vi "Target CSM.vi"(5 "Init State(\"Macro: Initialize\")":string="Macro: Initialize", 7 "Name(\"\" to use uuid)":string="CSM Tiny") -> ()   [LabVIEW 2017]
doc: "Template for building CSM Module without User Interface.\n\n<b>Inputs:</b>\n- <b>Name(\"\" to use uuid)</b>: Module Name\n - If Input is \"\", an uuid will be used for module name. The module is marked as stand-alone mode and will not be included in module list.\n - Fi Input end with '#', the module will worked in worker mode. Modules with the same name will shared the same message queue. Any external message will be processed by one of the modules, depends on who is free.\n - Otherwise, the input string will be used as module name, which should be unique in system. CSM will go to \"Critical Error\" state if duplicated module name is used in system.\n\n<b>Outputs:</b>\n - N/A"
uses:
  src/user.lib/_NEVSTOP/Communicable State Machine(CSM)/AdvanceAPI/CSM - Revert Arguments-Safe String.vi
  src/user.lib/_NEVSTOP/Communicable State Machine(CSM)/_Support/Common/Trim Single line Text.vi
  src/user.lib/_NEVSTOP/Communicable State Machine(CSM)/AdvanceAPI/CSM - Break Down Multiple States String.vi
  src/user.lib/_NEVSTOP/Communicable State Machine(CSM)/AdvanceAPI/CSM - Compact Multiple States.vi
  src/user.lib/_NEVSTOP/Communicable State Machine(CSM)/AdvanceAPI/CSM - Make String Arguments Safe.vi
  src/user.lib/_NEVSTOP/Communicable State Machine(CSM)/_Support/Common/Format Timestamp.vi
  src/user.lib/_NEVSTOP/Communicable State Machine(CSM)/AdvanceAPI/CSM - Keywords.vi
  src/user.lib/_NEVSTOP/Communicable State Machine(CSM)/Communicable State Machine.lvlib
panel:
  out "State History":string
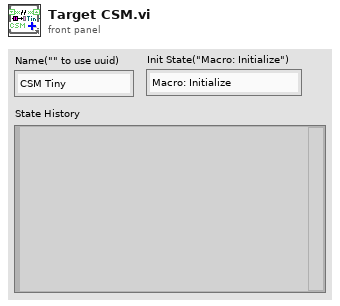
[diagram p1: front panel]
types:
  T1 = enum32{"Invalid", "Standard", "Closed", "Hidden", "Minimized", "Maximized"}
  T2 = enum32{"invalid app kind", "Development System", "Run Time System", "Student Edition", "Embedded LabVIEW", "Evaluation", "Custom"}
  T3 = typedef "Communicable State Machine.lvlib/_CSM_Response Source Message.ctl" = cluster{"‘State":string, "’Arguments":string, "’Error":errorcluster}
  T4 = cluster{"Core":cluster{"Current VI Reference":refnum<vi>, "Close Panel on Exit?":bool}, "Your Boolean data":bool, "Your string data":string}
  T5 = cluster{"Current VI Reference":refnum<vi>, "Close Panel on Exit?":bool}
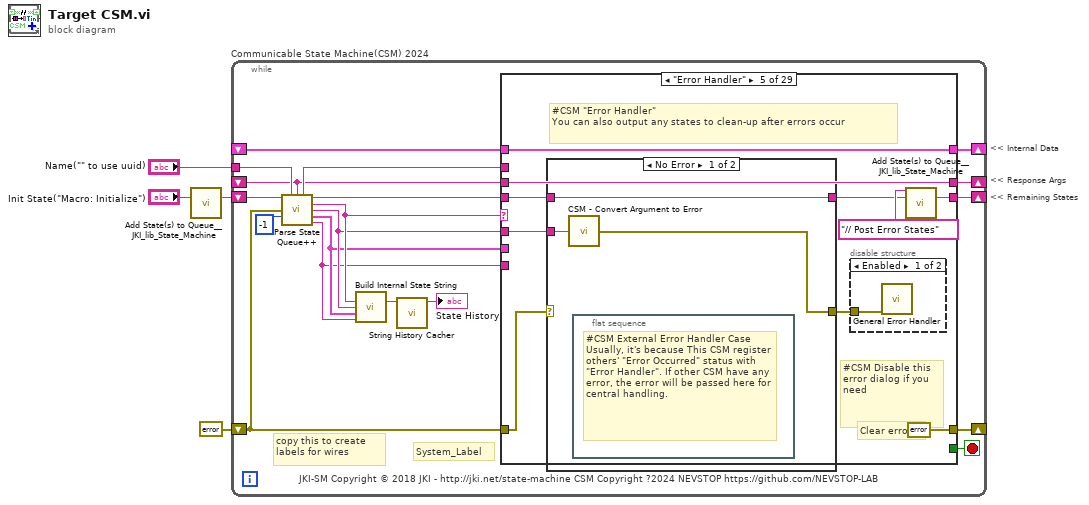
[diagram p0: block diagram]
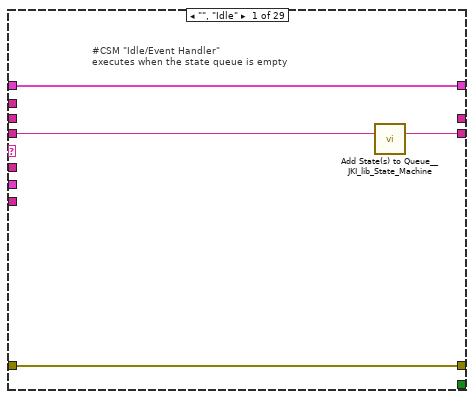
[diagram p2: hidden frame]
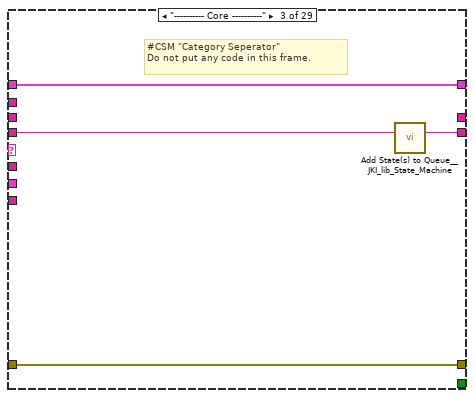
[diagram p4: hidden frame]
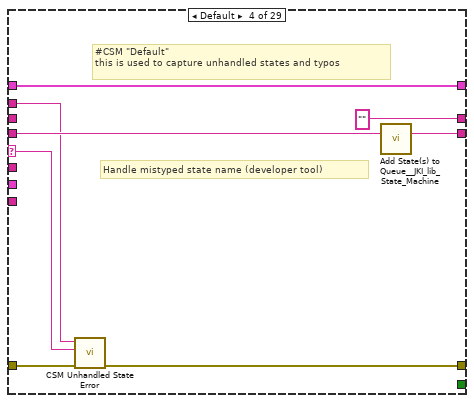
[diagram p5: hidden frame]
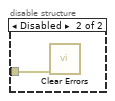
[diagram p6: hidden frame]
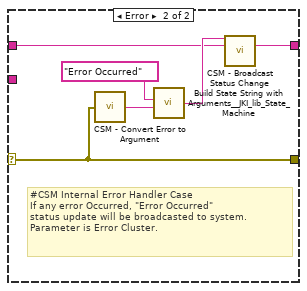
[diagram p7: hidden frame]
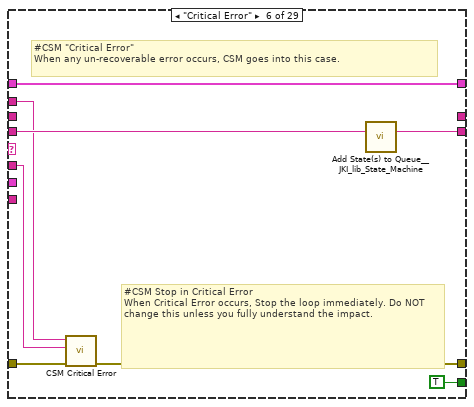
[diagram p8: hidden frame]
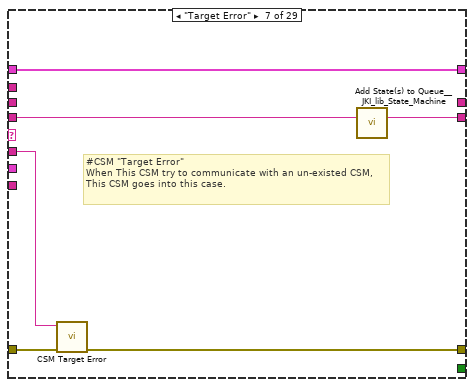
[diagram p9: hidden frame]
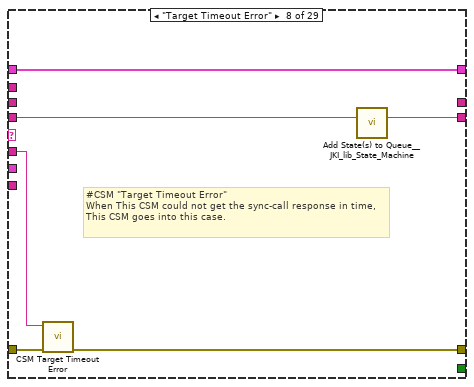
[diagram p10: hidden frame]
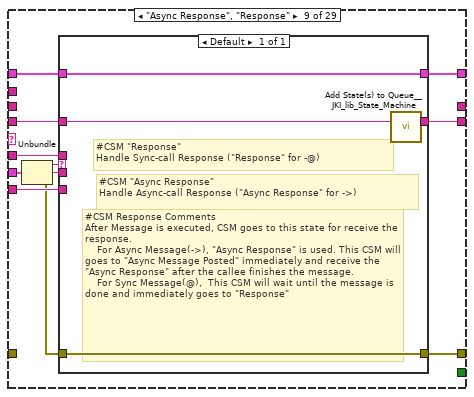
[diagram p11: hidden frame]
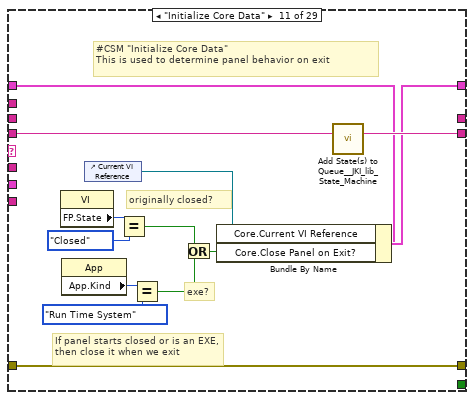
[diagram p13: hidden frame]
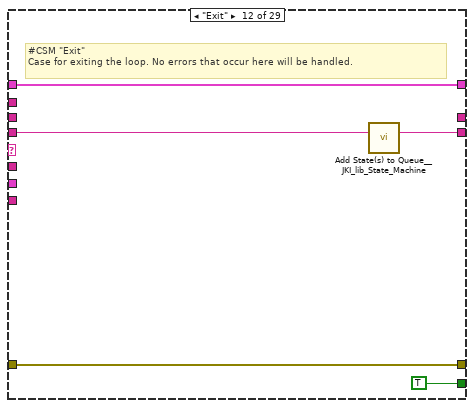
[diagram p14: hidden frame]
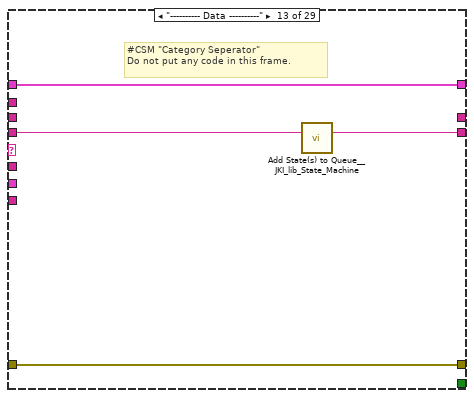
[diagram p15: hidden frame]
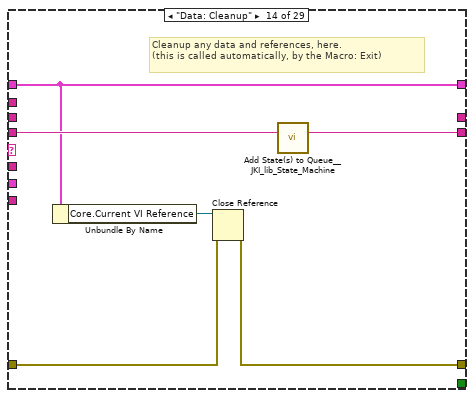
[diagram p16: hidden frame]
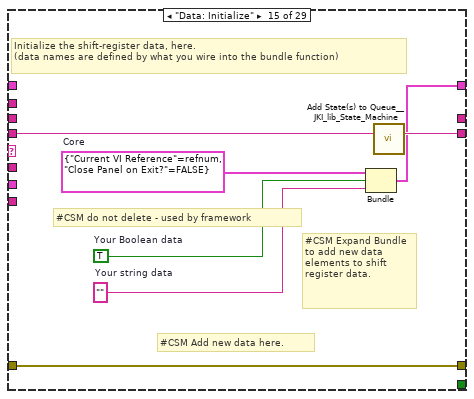
[diagram p17: hidden frame]
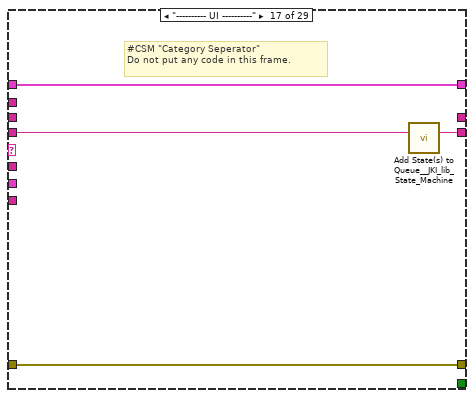
[diagram p19: hidden frame]
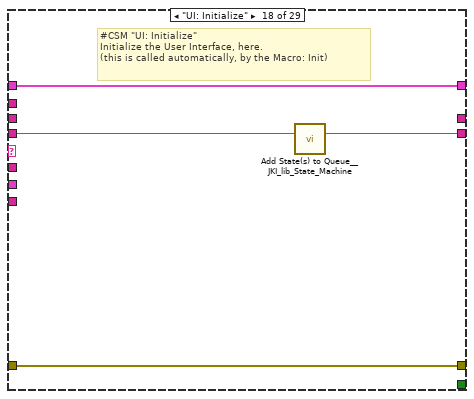
[diagram p20: hidden frame]
diagram:
  # "<< Internal Data"
  # "<< Response Args"
  # "<< Remaining States"
  n1 = call <vilib>:"Add State(s) to Queue__JKI_lib_State_Machine.vi"("State(s) in (\"\")"="Init State(\"Macro: Initialize\")") -> ("States Out"=w4:string)  [unwired: 14 in]
  n2 = while "Communicable State Machine(CSM) 2024" {
    shift-right: [w18] -> _
    shift-left: _ -> [w17]
    shift-right: [w21] -> _
    shift-left: errorcluster {"status"=FALSE, "code"=0, "source"=""} ("error out") -> [w16]
    shift-right: [w20] -> _
    shift-left: w4 -> [w22]
    tunnel: "Name(\"\" to use uuid)" -> [w14]
    shift-right: [w15] -> _
    shift-left: _ -> [w6]
    stop <- w19 stop-if-true
    # "copy this to create labels for wires"
    # "System_Label"
    # "JKI-SM Copyright © 2018 JKI - http://jki.net/state-machine CSM Copyright ?2024 NEVSTOP https://github.com/NEVSTOP-LAB"
    n3 = call "Parse State Queue++.vi"("State Queue"=w22, "Name(\"\" to use uuid)"=w14, "Response Arguments"=w6, "Error In (no error)"=w16, "Dequeue Timeout(0ms)"=-1 ("Timeout")) -> ("Name Used"=w7:string, "Remaining States"=w23:string, "Current State"=w11:string, "Arguments"=w10:string, ">> Response Source Message >>"=w9:T3, ">> Source CSM >>"=w8:string)  [unwired: 5 in]
    n4 = call "Build Internal State String.vi"("State"=w11, "Arguments (\"\")"=w10, ">> Response Source Message >>"=w9, "Source (\"\")"=w8) -> ("State with Arguments"=w12:string)  [unwired: 11 in]
    n5 = call "String History Cacher.vi"("String"=w12) -> ("String Cache"=→"State History":string)  [unwired: 10 in]
    n6 = case shown="\"Error Handler\"" w11 {
      selector: w11 -> [_ _ _ w37 _ _ _ _ _ _ _ _ _ _ _ _ _ _ _ _ _ _ _ _ _ _ _ _ _]
      tunnel: w23 -> [w24 w29 w34 w41 w48 w69 w75 w81 w89 w100 w114 w119 w123 w129 w136 w138 w143 w147 w153 w168 w237 w242 w249 w251 w256 w262 w267 w271 w275]
      tunnel: w10 -> [_ _ _ _ w47 w65 w74 w79 w88 _ _ _ _ _ _ _ _ _ w148 w162 _ _ _ _ w254 _ _ _ _]
      tunnel: w17 -> [w25 w28 w31 w39 w51 w70 w76 w82 w91 w99 w107 w117 w120 w124 _ w137 w140 w145 w151 w164 w234 w239 w246 w250 w255 w261 w264 w268 w272]
      tunnel: [w26 w30 w32 w35 errorcluster {"status"=FALSE, "code"=0, "source"=""} ("error out") w66 w72 w78 w94 w101 w111 w116 w121 w125 w133 w139 w141 w144 w149 w165 w235 w240 w247 w252 w257 w263 w265 w269 w273] -> w21
      tunnel: w16 -> [w26 w30 w32 w42 w49 w71 w73 w80 _ w101 w111 w116 w121 w126 w133 w139 w141 w144 w150 w166 w235 w240 w247 w252 w257 w263 w265 w269 w273]
      tunnel: [w27 w29 w33 w40 w44 w68 w77 w83 w90 w100 w113 w118 w122 w128 w135 w138 w142 w146 w152 w167 w236 w241 w248 w251 w256 w262 w266 w270 w274] -> w20
      tunnel: [_ _ _ _ _ TRUE _ _ _ _ _ TRUE _ _ _ _ _ _ _ _ _ _ _ _ _ _ _ _ _] -> w19
      tunnel: [w25 w28 w31 w39 w51 w70 w76 w82 w92 w99 w112 w117 w120 w124 w134 w137 w140 w145 w151 w164 w234 w239 w246 w250 w255 w261 w264 w268 w272] -> w18
      tunnel: w8 -> [_ _ _ _ _ _ _ _ w86 _ _ _ _ _ _ _ _ _ _ _ _ _ _ _ _ _ _ _ _]
      tunnel: w9 -> [_ _ _ _ _ _ _ _ w93 _ _ _ _ _ _ _ _ _ _ _ _ _ _ _ _ _ _ _ _]
      tunnel: [_ _ _ "" w43 _ _ _ _ _ _ _ _ _ _ _ _ _ _ _ _ _ _ _ w253 "API1 Response" _ _ _] -> w15
      tunnel: w7 -> [_ _ _ w36 _ w64 _ _ _ _ _ _ _ _ _ _ _ _ _ _ _ _ _ _ _ _ _ _ _]
      tunnel: w6 -> [_ _ _ _ w43 _ _ _ _ _ _ _ _ _ _ _ _ _ _ _ _ _ _ _ _ _ _ _ _]
      frame "", "Idle" {
        # "#CSM \"Idle/Event Handler\"\nexecutes when the state queue is empty"
        n7 = call <vilib>:"Add State(s) to Queue__JKI_lib_State_Machine.vi"("State(s) in (\"\")"=w24) -> ("States Out"=w27:string)  [unwired: 14 in]
      }
      frame "CSM Documentation" {
        # "#CSM README FIRST\n\nCommunicable State Machine(CSM) is a LabVIEW application framework that builds upon JKI State Machine(JKISM). It follows the pattern of JKISM and extends the keywords to describe message communication between modules, including concepts such as Sync-Message, Async-Message, Subscription/Unsubscription of status - essential elements for creating reusable code modules. For more information, please visit the CSM wiki: https://nevstop-lab.github.io/CSM-Wiki/\n\nFor instructions on JKI State Machine, visit: http://jki.net/state-machine/\nFor information about CSM, visit: https://github.com/NEVSTOP-LAB"
        # "#CSM \"Documentation\"\nCase for holding CSM Documenation"
      }
      frame "---------- Core ----------" {
        # "#CSM \"Category Seperator\"\nDo not put any code in this frame."
        n8 = call <vilib>:"Add State(s) to Queue__JKI_lib_State_Machine.vi"("State(s) in (\"\")"=w34) -> ("States Out"=w33:string)  [unwired: 14 in]
      }
      frame Default {
        # "#CSM \"Default\"\nthis is used to capture unhandled states and typos"
        # "Handle mistyped state name (developer tool)"
        n9 = call "CSM Unhandled State Error.vi"("error in (no error)"=w42, "Current State"=w37, "CSM Name"=w36) -> ("error out"=w35:errorcluster)  [unwired: 8 in]
        n10 = call <vilib>:"Add State(s) to Queue__JKI_lib_State_Machine.vi"("State(s) in (\"\")"=w41) -> ("States Out"=w40:string)  [unwired: 14 in]
      }
      frame "Error Handler" {
        # "#CSM Disable this error dialog if you need"
        # "#CSM \"Error Handler\"\nYou can also output any states to clean-up after errors occur"
        # "Clear error"
        n11 = case shown="No Error" w49 {
          selector: w49 -> [_ w58]
          tunnel: [w57 w60] -> w45
          tunnel: w48 -> [w57 w59]
          tunnel: w47 -> [w56 _]
          tunnel: [w55 w58] -> w50
          frame No Error {
            n12 = call "CSM - Convert Argument to Error.vi"("Argument"=w56) -> ("error"=w55:errorcluster)  [unwired: 4 in]
            n13 = flat-sequence {
              frame #0 {
                # "#CSM External Error Handler Case\nUsually, it's because This CSM register others' \"Error Occurred\" status with \"Error Handler\". If other CSM have any error, the error will be passed here for central handling."
              }
            }
          }
          frame Error {
            # "#CSM Internal Error Handler Case \nIf any error Occurred, \"Error Occurred\" \nstatus update will be broadcasted to system.\nParameter is Error Cluster."
            n14 = call "CSM - Convert Error to Argument.vi"("error in (no error)"=w58) -> ("Arguments"=w62:string)  [unwired: 4 in]
            n15 = call <vilib>:"Build State String with Arguments__JKI_lib_State_Machine.vi"("Arguments (\"\")"=w62, "State"="Error Occurred" ("Status with Arguments")) -> ("State with Arguments"=w61:string)  [unwired: 4 in]
            n16 = call "CSM - Broadcast Status Change.vi"("Status with Arguments"=w61, "State Queue"=w59) -> ("Remaining States"=w60:string)  [unwired: 13 in]
          }
        }
        n17 = disable-structure shown="Enabled" {
          disable-tunnel: w50 -> [w53 w54]
          frame Enabled {
            n18 = call <vilib>:"General Error Handler.vi"("error in (no error)"=w53) -> ()  [unwired: 10 in, 5 out]
          }
          frame Disabled {
            n19 = call <vilib>:"Clear Errors.vi"("error in (no error)"=w54) -> ()  [unwired: 5 in, 2 out]
          }
        }
        n20 = call <vilib>:"Add State(s) to Queue__JKI_lib_State_Machine.vi"("State(s) in Front (\"\")"="// Post Error States", "State(s) in (\"\")"=w45) -> ("States Out"=w44:string)  [unwired: 13 in]
      }
      frame "Critical Error" {
        # "#CSM Stop in Critical Error\nWhen Critical Error occurs, Stop the loop immediately. Do NOT change this unless you fully understand the impact."
        # "#CSM \"Critical Error\"\nWhen any un-recoverable error occurs, CSM goes into this case."
        n21 = call "CSM Critical Error.vi"("error in (no error)"=w71, "Arugments(as Reason)"=w65, "CSM Name"=w64) -> ("error out"=w66:errorcluster)  [unwired: 8 in]
        n22 = call <vilib>:"Add State(s) to Queue__JKI_lib_State_Machine.vi"("State(s) in (\"\")"=w69) -> ("States Out"=w68:string)  [unwired: 14 in]
      }
      frame "Target Error" {
        # "#CSM \"Target Error\"\nWhen This CSM try to communicate with an un-existed CSM, This CSM goes into this case."
        n23 = call "CSM Target Error.vi"("error in (no error)"=w73, "Arguments(as CSM Name)"=w74) -> ("error out"=w72:errorcluster)  [unwired: 9 in]
        n24 = call <vilib>:"Add State(s) to Queue__JKI_lib_State_Machine.vi"("State(s) in (\"\")"=w75) -> ("States Out"=w77:string)  [unwired: 14 in]
      }
      frame "Target Timeout Error" {
        # "#CSM \"Target Timeout Error\"\nWhen This CSM could not get the sync-call response in time, This CSM goes into this case."
        n25 = call "CSM Target Timeout Error.vi"("error in (no error)"=w80, "Arguments(as CSM Name)"=w79) -> ("error out"=w78:errorcluster)  [unwired: 9 in]
        n26 = call <vilib>:"Add State(s) to Queue__JKI_lib_State_Machine.vi"("State(s) in (\"\")"=w81) -> ("States Out"=w83:string)  [unwired: 14 in]
      }
      frame "Async Response", "Response" {
        n27 = Unbundle(w93) -> ("‘State"=w87:string, "’Arguments"=w85:string, "’Error"=w84:errorcluster)
        n28 = case shown="Default" w87 {
          tunnel: [w98] -> w94
          tunnel: w84 -> [w98]
          tunnel: [w97] -> w92
          tunnel: w91 -> [w97]
          tunnel: [w95] -> w90
          tunnel: w89 -> [w96]
          tunnel: w88 -> [_]
          tunnel: w86 -> [_]
          tunnel: w85 -> [_]
          frame Default {
            # "#CSM Response Comments\nAfter Message is executed, CSM goes to this state for receive the response.\n    For Async Message(->), \"Async Response\" is used. This CSM will goes to \"Async Message Posted\" immediately and receive the \"Async Response\" after the callee finishes the message.\n    For Sync Message(@),  This CSM will wait until the message is done and immediately goes to \"Response\""
            # "#CSM \"Async Response\"\nHandle Async-call Response (\"Async Response\" for ->)"
            # "#CSM \"Response\"\nHandle Sync-call Response (\"Response\" for -@)"
            n29 = call <vilib>:"Add State(s) to Queue__JKI_lib_State_Machine.vi"("State(s) in (\"\")"=w96) -> ("States Out"=w95:string)  [unwired: 14 in]
          }
        }
      }
      frame "Async Message Posted" {
        # "a"
        # "a"
        # "a"
        # "a"
        # "a"
        # "a"
        # "a"
        # "a"
        # "a"
        # "a"
        # "a"
        # "a"
        # "a"
        # "a"
        # "a"
        # "a"
        # "a"
        # "a"
        # "a"
        # "a"
        # "a"
        # "a"
        # "a"
        # "a"
        # "a"
        # "a"
        # "a"
        # "a"
        # "a"
        # "a"
        # "a"
        # "a"
        # "a"
        # "a"
        # "a"
        # "a"
        # "a"
        # "a"
        # "a"
        # "a"
        # "a"
        # "a"
        # "a"
        # "a"
        # "a"
        # "a"
        # "a"
        # "a"
        # "a"
        # "a"
        # "a"
        # "a"
        # "a"
        # "a"
        # "a"
        # "a"
        # "a"
        # "a"
        # "a"
        # "a"
        # "a"
        # "a"
        # "a"
        # "a"
        # "a"
        # "a"
        # "a"
        # "a"
        # "a"
        # "a"
        # "a"
        # "a"
        # "a"
        # "a"
        # "a"
        # "a"
        # "a"
        # "a"
        # "a"
        # "a"
        # "a"
        # "a"
        # "a"
        # "a"
        # "a"
        # "a"
        # "a"
        # "a"
        # "a"
        # "a"
        # "a"
        # "a"
        # "a"
        # "a"
        # "a"
        # "a"
        # "a"
        # "a"
        # "a"
        # "a"
        # "a"
        # "a"
        # "a"
        # "a"
        # "a"
        # "a"
        # "a"
        # "a"
        # "a"
        # "a"
        # "a"
        # "a"
        # "a"
        # "a"
        # "a"
        # "a"
        # "a"
        # "a"
        # "a"
        # "a"
        # "a"
        # "a"
        # "a"
        # "a"
        # "a"
        # "a"
        # "a"
        # "a"
        # "a"
        # "a"
        # "a"
        # "a"
        # "a"
        # "a"
        # "a"
        # "a"
        # "a"
        # "a"
        # "a"
        # "a"
        # "a"
        # "a"
        # "a"
        # "a"
        # "a"
        # "a"
        # "a"
        # "a"
        # "a"
        # "a"
        # "a"
        # "a"
        # "a"
        # "a"
        # "a"
        # "a"
        # "a"
        # "a"
        # "a"
        # "a"
        # "a"
        # "a"
        # "a"
        # "a"
        # "a"
        # "a"
        # "a"
        # "a"
        # "a"
        # "a"
        # "a"
        # "a"
        # "a"
        # "a"
        # "a"
        # "a"
        # "a"
        # "a"
        # "a"
        # "a"
        # "a"
        # "a"
        # "a"
        # "a"
        # "a"
        # "a"
        # "a"
        # "a"
        # "a"
        # "a"
        # "a"
        # "a"
        # "a"
        # "a"
        # "a"
        # "a"
        # "a"
        # "a"
        # "a"
        # "a"
        # "a"
        # "a"
        # "a"
        # "a"
        # "a"
        # "a"
        # "a"
        # "a"
        # "a"
        # "a"
        # "a"
        # "a"
        # "a"
        # "a"
        # "a"
        # "a"
        # "a"
        # "a"
        # "a"
        # "a"
        # "a"
        # "a"
        # "a"
        # "a"
        # "a"
        # "a"
        # "a"
        # "a"
        # "a"
        # "a"
        # "a"
        # "a"
        # "a"
        # "a"
        # "a"
        # "a"
        # "a"
        # "a"
        # "a"
        # "a"
        # "a"
        # "a"
        # "a"
        # "a"
        # "a"
        # "a"
        # "a"
        # "a"
        # "a"
        # "a"
        # "a"
        # "a"
        # "a"
        # "a"
        # "a"
        # "a"
        # "a"
        # "a"
        # "a"
        # "a"
        # "a"
        # "a"
        # "a"
        # "a"
        # "a"
        # "a"
        # "a"
        # "a"
        # "a"
        # "a"
        # "a"
        # "a"
        # "a"
        # "a"
        # "a"
        # "a"
        # "a"
        # "a"
        # "a"
        # "a"
        # "a"
        # "a"
        # "a"
        # "a"
        # "a"
        # "a"
        # "a"
        # "a"
        # "a"
        # "a"
        # "a"
        # "a"
        # "a"
        # "a"
        # "a"
        # "a"
        # "a"
        # "a"
        # "a"
        # "a"
        # "a"
        # "a"
        # "a"
        # "a"
        # "a"
        # "a"
        # "a"
        # "a"
        # "a"
        # "a"
        # "a"
        # "a"
        # "a"
        # "a"
        # "a"
        # "a"
        # "a"
        # "a"
        # "a"
        # "a"
        # "a"
        # "a"
        # "a"
        # "a"
        # "a"
        # "a"
        # "a"
        # "a"
        # "a"
        # "a"
        # "a"
        # "a"
        # "a"
        # "a"
        # "a"
        # "a"
        # "a"
        # "a"
        # "a"
        # "a"
        # "a"
        # "a"
        # "a"
        # "a"
        # "a"
        # "a"
        # "a"
        # "a"
        # "a"
        # "a"
        # "a"
        # "a"
        # "a"
        # "a"
        # "a"
        # "a"
        # "a"
        # "a"
        # "a"
        # "a"
        # "a"
        # "a"
        # "a"
        # "a"
        # "a"
        # "a"
        # "a"
        # "a"
        # "a"
        # "a"
        # "a"
        # "a"
        # "a"
        # "a"
        # "a"
        # "a"
        # "a"
        # "a"
      }
      frame "Initialize Core Data" {
        # "#CSM \"Initialize Core Data\"\nThis is used to determine panel behavior on exit"
        # "originally closed?"
        # "exe?"
        # "If panel starts closed or is an EXE, then close it when we exit"
        n30 = property class="VI"() -> ("FP.State"=w104:T1)  [unwired: 2 in, 2 out]
        n31 = property class="App"() -> ("App.Kind"=w110:T2)  [unwired: 2 in, 2 out]
        n32 = control-ref of="Current VI Reference"() -> (w105:refnum<vi>)
        n33 = Equal?(x=w104, y=T1."Closed" ("Front Panel Window:State")) -> (x = y?=w102:bool)
        n34 = Equal?(x=w110, y=T2."Run Time System" ("Application:Kind")) -> (x = y?=w108:bool)
        n35 = Or(x=w102, y=w108) -> (x .or. y?=w106:bool)
        n36 = Bundle By Name(cluster=w107, "Core.Current VI Reference"=w105, "Core.Close Panel on Exit?"=w106) -> (w112:T4)
        n37 = call <vilib>:"Add State(s) to Queue__JKI_lib_State_Machine.vi"("State(s) in (\"\")"=w114) -> ("States Out"=w113:string)  [unwired: 14 in]
      }
      frame "Exit" {
        # "#CSM \"Exit\"\nCase for exiting the loop. No errors that occur here will be handled."
        n38 = call <vilib>:"Add State(s) to Queue__JKI_lib_State_Machine.vi"("State(s) in (\"\")"=w119) -> ("States Out"=w118:string)  [unwired: 14 in]
      }
      frame "---------- Data ----------" {
        # "#CSM \"Category Seperator\"\nDo not put any code in this frame."
        n39 = call <vilib>:"Add State(s) to Queue__JKI_lib_State_Machine.vi"("State(s) in (\"\")"=w123) -> ("States Out"=w122:string)  [unwired: 14 in]
      }
      frame "Data: Cleanup" {
        # "Cleanup any data and references, here.\n(this is called automatically, by the Macro: Exit)"
        n40 = Unbundle By Name(w124) -> ("Core.Current VI Reference"=w127:refnum<vi>)
        n41 = Close Reference(reference=w127, error in (no error)=w126) -> (error out=w125:errorcluster)
        n42 = call <vilib>:"Add State(s) to Queue__JKI_lib_State_Machine.vi"("State(s) in (\"\")"=w129) -> ("States Out"=w128:string)  [unwired: 14 in]
      }
      frame "Data: Initialize" {
        w130 = T5 {"Current VI Reference"=refnum, "Close Panel on Exit?"=FALSE}  # Core
        w132 = TRUE  # Your Boolean data
        w131 = ""  # Your string data
        # "#CSM do not delete - used by framework"
        # "#CSM Expand Bundle to add new data elements to shift register data."
        # "#CSM Add new data here."
        # "Initialize the shift-register data, here.\n(data names are defined by what you wire into the bundle function)"
        n43 = Bundle("Core"=w130, "Your Boolean data"=w132, "Your string data"=w131) -> (w134:T4)  [unwired: 1 in]
        n44 = call <vilib>:"Add State(s) to Queue__JKI_lib_State_Machine.vi"("State(s) in (\"\")"=w136) -> ("States Out"=w135:string)  [unwired: 14 in]
      }
      frame "Data: Update Indicators" {
      }
      frame "---------- UI ----------" {
        # "#CSM \"Category Seperator\"\nDo not put any code in this frame."
        n45 = call <vilib>:"Add State(s) to Queue__JKI_lib_State_Machine.vi"("State(s) in (\"\")"=w143) -> ("States Out"=w142:string)  [unwired: 14 in]
      }
      frame "UI: Initialize" {
        # "#CSM \"UI: Initialize\"\nInitialize the User Interface, here.\n(this is called automatically, by the Macro: Init)"
        n46 = call <vilib>:"Add State(s) to Queue__JKI_lib_State_Machine.vi"("State(s) in (\"\")"=w147) -> ("States Out"=w146:string)  [unwired: 14 in]
      }
      frame "UI: Cursor Set" {
        # "#CSM \"UI: Cursor Set\"\nSet and Unset Cursor Busy.\n(Usage: \"UI: Cursor Set >> Busy|Idle\")"
        # "Argument"
        n47 = disable-structure shown="TARGET_TYPE!=Windows" {
          disable-tunnel: w150 -> [w156 w161]
          disable-tunnel: [w155 w161] -> w149
          disable-tunnel: w148 -> [w154 _]
          frame condition #0 (active) {
            n48 = case shown="\"Idle\", Default" w154 {
              tunnel: w156 -> [w158 w160]
              tunnel: [w157 w159] -> w155
              frame "Idle", Default {
                n49 = call <vilib>:"Unset Busy.vi"("error in (no error)"=w158) -> ("error out"=w157:errorcluster)  [unwired: 10 in]
              }
              frame "Busy" {
                n50 = call <vilib>:"Set Busy.vi"("error in (no error)"=w160) -> ("error out"=w159:errorcluster)  [unwired: 9 in, 1 out]
              }
            }
          }
          frame condition #1 {
          }
        }
        n51 = call <vilib>:"Add State(s) to Queue__JKI_lib_State_Machine.vi"("State(s) in (\"\")"=w153) -> ("States Out"=w152:string)  [unwired: 14 in]
      }
      frame "UI: Front Panel State" {
        # "#CSM \"UI: Front Panel State\"\nSet Front Panel Open or Closed\n(Usage: \"UI: Front Panel State >> Open|Close\")"
        # "Argument"
        n52 = Unbundle By Name(w164) -> ("Core.Current VI Reference"=w163:refnum<vi>)
        n53 = call <vilib>:"Add State(s) to Queue__JKI_lib_State_Machine.vi"("State(s) in (\"\")"=w168) -> ("States Out"=w167:string)  [unwired: 14 in]
        n54 = case shown="\"Close\", \"Closed\"" w162 {
          tunnel: w166 -> [w174 w189 w200 w213 w226]
          tunnel: [w176 w190 w202 w215 w228] -> w165
          tunnel: w163 -> [w175 w187 w201 w214 w227]
          frame "Open", "Standard", Default {
            w169 = T1."Standard" ("State")
            n55 = property class="VI"(reference=w175, error in=w174) -> (reference out=w172:refnum<vi>, error out=w173:errorcluster, "FP.State"=w171:T1)
            n56 = Not Equal?(x=w171, y=w169) -> (x != y?=w170:bool)
            n57 = case shown="True" w170 {
              tunnel: [w180 w182] -> w176
              tunnel: w173 -> [w179 w182]
              tunnel: w172 -> [w178 _]
              tunnel: w169 -> [w177 _]
              frame True {
                n58 = invoke class="VI" method="FP.Open"(reference=w178, error in=w179, "Activate"=TRUE, "State"=w177) -> (error out=w180:errorcluster)  [unwired: 1 in, 4 out]
              }
              frame False {
              }
            }
          }
          frame "Close", "Closed" {
            n59 = property class="VI"(reference=w187, error in=w189) -> (reference out=w186:refnum<vi>, error out=w188:errorcluster, "FP.State"=w184:T1)
            n60 = Not Equal?(x=w184, y=T1."Closed" ("Front Panel Window:State")) -> (x != y?=w183:bool)
            n61 = case shown="False" w183 {
              tunnel: [w191 w194] -> w190
              tunnel: w188 -> [w191 w193]
              tunnel: w186 -> [_ w192]
              frame False {
              }
              frame True {
                n62 = invoke class="VI" method="FP.Close"(reference=w192, error in=w193) -> (error out=w194:errorcluster)  [unwired: 1 in, 2 out]
              }
            }
          }
          frame "Hidden", "Hide" {
            w195 = T1."Hidden" ("State")
            n63 = property class="VI"(reference=w201, error in=w200) -> (reference out=w198:refnum<vi>, error out=w199:errorcluster, "FP.State"=w197:T1)
            n64 = Not Equal?(x=w197, y=w195) -> (x != y?=w196:bool)
            n65 = case shown="True" w196 {
              tunnel: [w206 w207] -> w202
              tunnel: w199 -> [w205 w207]
              tunnel: w198 -> [w204 _]
              tunnel: w195 -> [w203 _]
              frame True {
                n66 = invoke class="VI" method="FP.Open"(reference=w204, error in=w205, "State"=w203) -> (error out=w206:errorcluster)  [unwired: 2 in, 4 out]
              }
              frame False {
              }
            }
          }
          frame "Minimize", "Minimized" {
            w208 = T1."Minimized" ("State")
            n67 = property class="VI"(reference=w214, error in=w213) -> (reference out=w211:refnum<vi>, error out=w212:errorcluster, "FP.State"=w210:T1)
            n68 = Not Equal?(x=w210, y=w208) -> (x != y?=w209:bool)
            n69 = case shown="True" w209 {
              tunnel: [w219 w220] -> w215
              tunnel: w212 -> [w218 w220]
              tunnel: w211 -> [w217 _]
              tunnel: w208 -> [w216 _]
              frame True {
                n70 = invoke class="VI" method="FP.Open"(reference=w217, error in=w218, "State"=w216) -> (error out=w219:errorcluster)  [unwired: 2 in, 4 out]
              }
              frame False {
              }
            }
          }
          frame "Maximize", "Maximized" {
            w221 = T1."Maximized" ("State")
            n71 = property class="VI"(reference=w227, error in=w226) -> (reference out=w224:refnum<vi>, error out=w225:errorcluster, "FP.State"=w223:T1)
            n72 = Not Equal?(x=w223, y=w221) -> (x != y?=w222:bool)
            n73 = case shown="True" w222 {
              tunnel: [w232 w233] -> w228
              tunnel: w225 -> [w231 w233]
              tunnel: w224 -> [w230 _]
              tunnel: w221 -> [w229 _]
              frame True {
                n74 = invoke class="VI" method="FP.Open"(reference=w230, error in=w231, "State"=w229) -> (error out=w232:errorcluster)  [unwired: 2 in, 4 out]
              }
              frame False {
              }
            }
          }
        }
      }
      frame "---------- Macro ----------" {
        # "#CSM \"Category Seperator\"\nDo not put any code in this frame."
        n75 = call <vilib>:"Add State(s) to Queue__JKI_lib_State_Machine.vi"("State(s) in (\"\")"=w237) -> ("States Out"=w236:string)  [unwired: 14 in]
      }
      frame "Macro: Initialize" {
        # "#CSM \"Macro: Initialize\"\nInitialization Macro (This is called once, when the VI starts)"
        n76 = call <vilib>:"Add State(s) to Queue__JKI_lib_State_Machine.vi"("State(s) in Front (\"\")"="Data: Initialize\nInitialize Core Data\nData: Update Indicators", "State(s) in (\"\")"=w242) -> ("States Out"=w241:string)  [unwired: 13 in]
      }
      frame "Macro: Exit" {
        # "#CSM \"Macro: Exit\"\nExit Macro (This is called once, when the VI exits)"
        n77 = call <vilib>:"Add State(s) to Queue__JKI_lib_State_Machine.vi"("State(s) in Front (\"\")"="//Exit Sub-Modules ", "State(s) at Back (\"\")"="Data: Cleanup\nExit") -> ("States Out"=w244:string)  [unwired: 13 in]
        n78 = call <vilib>:"Add State(s) to Queue__JKI_lib_State_Machine.vi"("State(s) in Front (\"\")"=w244, "State(s) in (\"\")"=w249) -> ("States Out"=w248:string)  [unwired: 13 in]
      }
      frame "---------- API ----------" {
        # "#CSM \"Category Seperator\"\nDo not put any code in this frame."
      }
      frame "API: API2" {
        # "#CSM API Example\nCopy/Rename this case for your own API"
        # "unpack Hex String  to Variant\nif complex parameter is needed."
        n79 = call "CSM - Convert HexStr to Data.vi"("HEX String"=w254) -> ()  [unwired: 7 in, 2 out]
        n80 = disable-structure shown="Disabled" {
          disable-tunnel: [w258 "API2 Response"] -> w253
          frame Disabled {
            # "pack variant to hexstr \nif complex response is needed."
            # "complex Response"
            n81 = call "CSM - Convert Data to HexStr.vi"() -> ("HEX String (0-9,A-F)"=w258:string)  [unwired: 9 in]
          }
          frame Enabled {
          }
        }
      }
      frame "API: API1" {
        # "#CSM API Example\nCopy/Rename this case for your own API"
        # "#CSM Response\nConnect this to return the response of your API"
        # "#CSM >> Source CSM >>\nIf you need to tell who triggered this state , use this string. If it's this case itself, this string is \"\"."
        # "#CSM >> Arguments >>\nDeal with the parameter if any"
      }
      frame "---------- Action ----------" {
        # "#CSM \"Category Seperator\"\nDo not put any code in this frame."
        n82 = call <vilib>:"Add State(s) to Queue__JKI_lib_State_Machine.vi"("State(s) in (\"\")"=w267) -> ("States Out"=w266:string)  [unwired: 14 in]
      }
      frame "Action: action1" {
        # "#CSM \"Internal State\"\nThis category is used for holding internal states"
        n83 = call <vilib>:"Add State(s) to Queue__JKI_lib_State_Machine.vi"("State(s) in (\"\")"=w271) -> ("States Out"=w270:string)  [unwired: 14 in]
      }
      frame "Action: action2" {
        # "#CSM \"Internal State\"\nThis category is used for holding internal states"
        n84 = call <vilib>:"Add State(s) to Queue__JKI_lib_State_Machine.vi"("State(s) in (\"\")"=w275) -> ("States Out"=w274:string)  [unwired: 14 in]
      }
    }
  }
